vi "test display resonance.vi"(11 "lines (2pi) per frame":i32) -> ()   [LabVIEW 2012]
panel:
  in  "Boolean":bool
  out "size(s) 2":i32[](array[numeric])
  out "x-y":u32
  in  "16-bit Display Mapping:All Elements":T1={"Conversion Method"=2, "Minimum Value"=-1000, "Maximum Value"=0, "Number Of Shifts"=0}
  out "error out":errorcluster
  out "Image":T2(plugin-control)
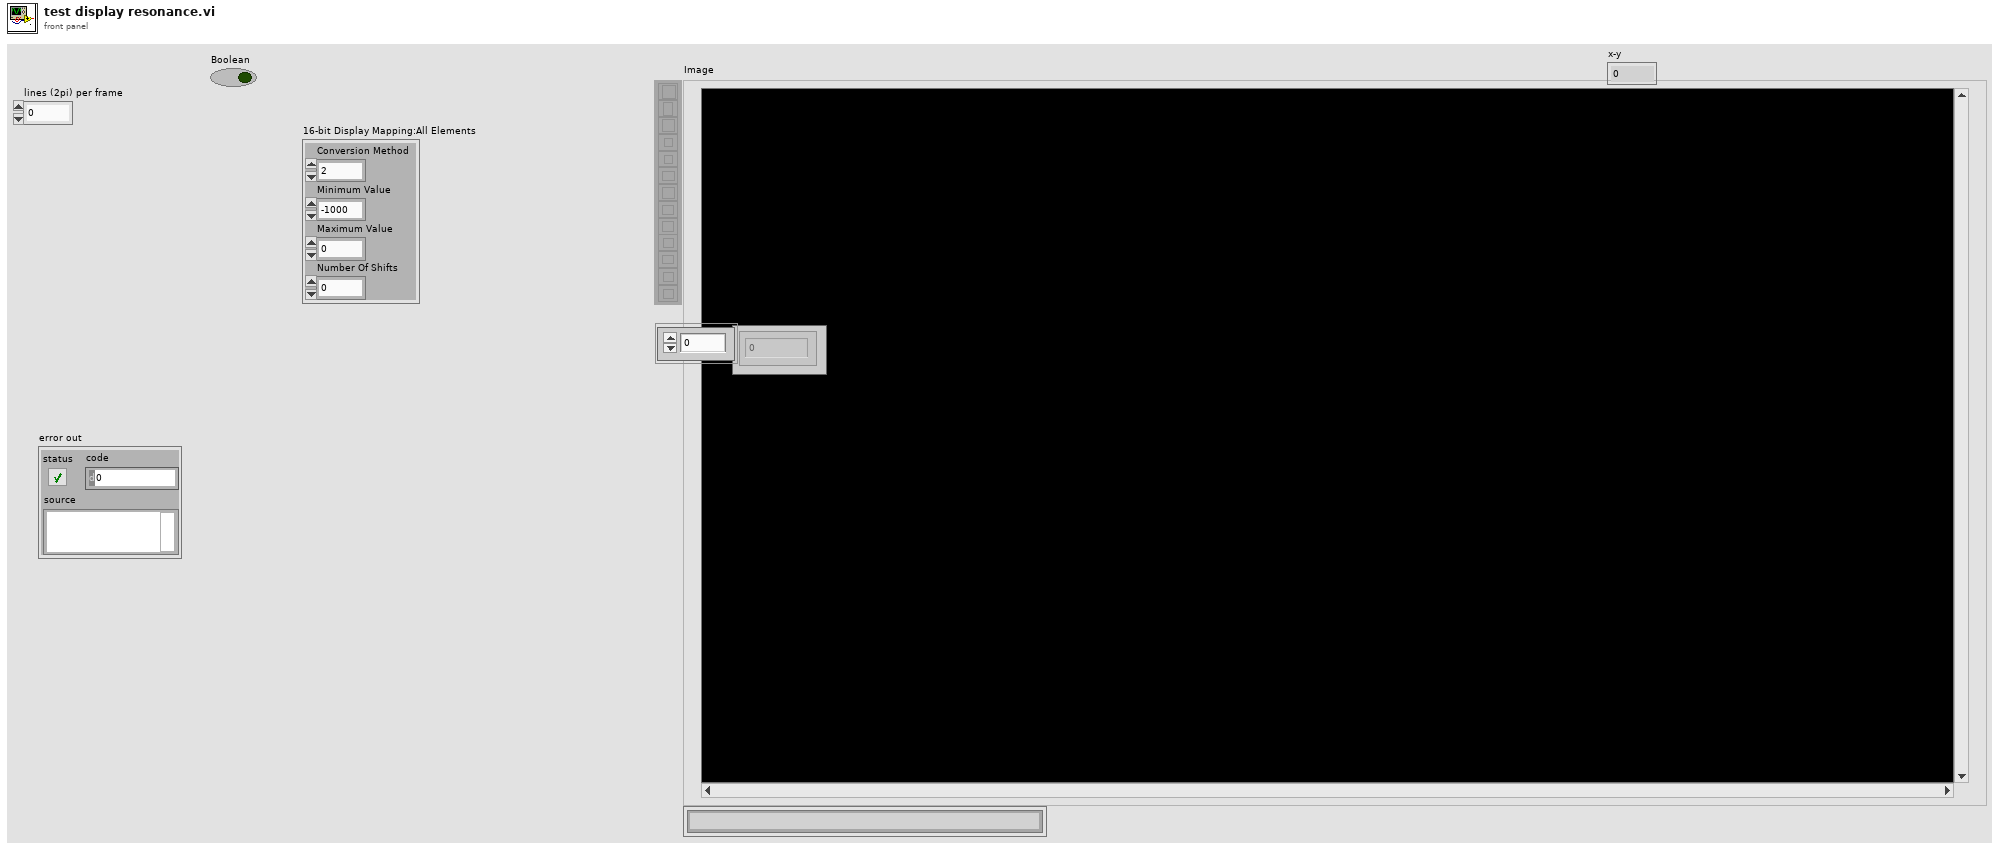
[diagram p1: front panel]
types:
  T1 = cluster{"Conversion Method":u32, "Minimum Value":i32, "Maximum Value":i32, "Number Of Shifts":i32}
  T2 = typedef "IMAQ Image.ctl" = refnum<image>
  T3 = typedef "Image Type" = u32
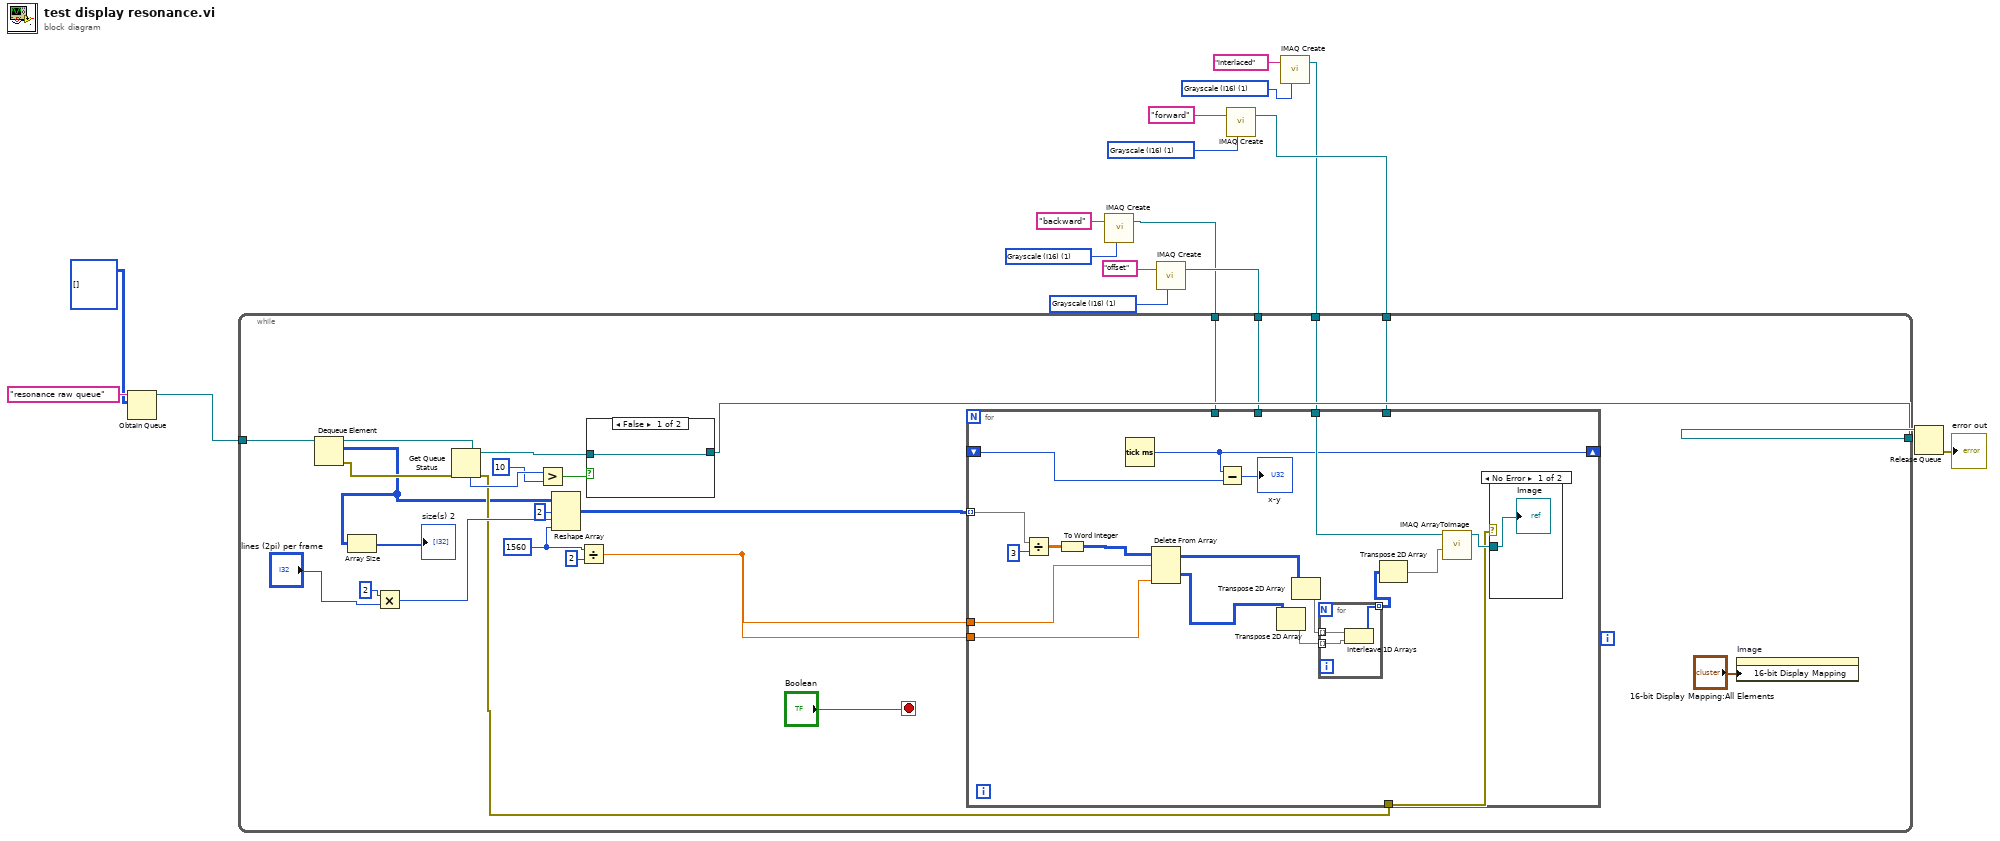
[diagram p0: block diagram]
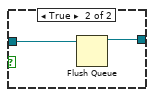
[diagram p2: hidden frame]
diagram:
  w13 = T3 1 items=["Grayscale (U8)", "Grayscale (I16)", "Grayscale (SGL)", "Complex (CSG)", "RGB (U32)", "HSL (U32)", "RGB (U64)", "Grayscale (U16)"] ("Image Type")
  w10 = T3 1 items=["Grayscale (U8)", "Grayscale (I16)", "Grayscale (SGL)", "Complex (CSG)", "RGB (U32)", "HSL (U32)", "RGB (U64)", "Grayscale (U16)"] ("Image Type")
  w9 = T3 1 items=["Grayscale (U8)", "Grayscale (I16)", "Grayscale (SGL)", "Complex (CSG)", "RGB (U32)", "HSL (U32)", "RGB (U64)", "Grayscale (U16)"] ("Image Type")
  w6 = T3 1 items=["Grayscale (U8)", "Grayscale (I16)", "Grayscale (SGL)", "Complex (CSG)", "RGB (U32)", "HSL (U32)", "RGB (U64)", "Grayscale (U16)"] ("Image Type")
  n1 = Obtain Queue(name (unnamed)="resonance raw queue", element data type=i32[][][] [] ("initialized array")) -> (queue out=w15:refnum<queue>)  [unwired: 3 in, 2 out]
  n2 = call "IMAQ Create"("Image Name"="backward", "Image Type"=w9) -> ("New Image"=w3:T2)  [unwired: 3 in, 1 out]
  n3 = call "IMAQ Create"("Image Name"="offset", "Image Type"=w10) -> ("New Image"=w4:T2)  [unwired: 3 in, 1 out]
  n4 = call "IMAQ Create"("Image Name"="forward", "Image Type"=w6) -> ("New Image"=w5:T2)  [unwired: 3 in, 1 out]
  n5 = call "IMAQ Create"("Image Name"="interlaced", "Image Type"=w13) -> ("New Image"=w1:T2)  [unwired: 3 in, 1 out]
  n6 = while {
    tunnel: w15 -> [w42]
    tunnel: [w39] -> w14
    tunnel: w5 -> [w38]
    tunnel: w4 -> [w37]
    tunnel: w3 -> [w36]
    tunnel: w1 -> [w35]
    stop <- "Boolean" stop-if-true
    w23 = 1560 ("dimension size")
    n7 = Dequeue Element(queue=w42) -> (queue out=w34:refnum<queue>, element=w19:i32[][][], error out=w29:errorcluster)  [unwired: 2 in, 1 out]
    n8 = Array Size(array=w19) -> (size(s)=→"size(s) 2":i32[])
    n9 = Multiply(x=2 ("dimension size"), y="lines (2pi) per frame") -> (x*y=w24:i32)
    n10 = Get Queue Status(queue=w34, error in (no error)=w29) -> (queue out=w33:refnum<queue>, error out=w22:errorcluster, # elements in queue=w32:i32)  [unwired: 1 in, 5 out]
    n11 = Greater?(x=w32, y=10) -> (0:w30:bool)
    n12 = Reshape Array(w19, 2 ("dimension size"), w24, w23) -> (w26:i32[][][])
    n13 = Divide(x=w23, y=2) -> (x/y=w21:dbl)
    n14 = case shown="False" w30 {
      tunnel: [w43 w45] -> w39
      tunnel: w33 -> [w43 w44]
      frame False {
      }
      frame True {
        n15 = Flush Queue(queue=w44) -> (queue out=w45:refnum<queue>)  [unwired: 1 in, 2 out]
      }
    }
    n16 = for {
      tunnel: w26 -> [w61] mode=indexing
      tunnel: w21 -> [w53]
      tunnel: w38 -> [_]
      tunnel: w37 -> [_]
      tunnel: w36 -> [_]
      tunnel: w35 -> [w60]
      shift-right: [w58] -> _
      shift-left: _ -> [w57]
      tunnel: w22 -> [w54]
      tunnel: w21 -> [w50]
      n17 = Divide(x=w61, y=3 ("element")) -> (x/y=w63:dbl[][])
      n18 = To Word Integer(number=w63) -> (16bit integer=w47:i16[][])
      n19 = Tick Count (ms)() -> (millisecond timer value=w58:u32)
      n20 = Delete From Array(array=w47, length=w53, index (col)=w50) -> (deleted portion=w46:i16[][], array with subset deleted=w49:i16[][])  [unwired: 1 in]
      n21 = Subtract(x=w58, y=w57) -> (x-y=→"x-y":u32)
      n22 = Transpose 2D Array(2D array=w46) -> (transposed array=w52:i16[][])
      n23 = Transpose 2D Array(2D array=w49) -> (transposed array=w51:i16[][])
      n24 = for {
        tunnel: w51 -> [w67] mode=indexing
        tunnel: w52 -> [w66] mode=indexing
        tunnel: [w65] -> w59 mode=indexing
        n25 = Interleave 1D Arrays(w67, w66) -> (w65:i16[])
      }
      n26 = Transpose 2D Array(2D array=w59) -> (transposed array=w48:i16[][])
      n27 = call "IMAQ ArrayToImage"("Image Pixels (I16)"=w48, "Image"=w60) -> ("Image Out"=w55:T2)  [unwired: 8 in, 1 out]
      n28 = case shown="No Error" w54 {
        tunnel: w55 -> [w64 _]
        frame No Error {
          "Image" <- w64
        }
        frame Error {
        }
      }
    }
    n29 = property on="Image" class="ImageControl"("16-bit Display Mapping"="16-bit Display Mapping:All Elements") -> ()  [unwired: 2 in, 2 out]
  }
  n30 = Release Queue(queue=w14) -> (error out=→"error out":errorcluster)  [unwired: 2 in, 2 out]
